vi ".....FACE RECOGNITION only.vi"() -> ()   [LabVIEW 2018]
doc: "This example shows how to use the Lucas Kanade Pyramid motion estimation VI to track features in a sequence of images in NI Vision. The VI reads the frames from an AVI file and tracks user specified features in the image from frame to frame."
uses:
  <vilib>/University of Leeds/Kinesthesia Toolkit for Microsoft Kinect/_Polymorphic Configure/Event-Video.vi
  <vilib>/University of Leeds/Kinesthesia Toolkit for Microsoft Kinect/_Polymorphic Read/Read-Video.vi
  <vilib>/University of Leeds/Kinesthesia Toolkit for Microsoft Kinect/_Polymorphic Close/Close-Video.vi
  <vilib>/vision/NI_Vision_Development_Module.lvlib
panel:
  out "Lips Template":T1(plugin-control)
  out "Nose Template":T1(plugin-control)
  out "Eye Template":T1(plugin-control)
  in  "Eye Min Score":sgl=700.0
  in  "Nose Min Score":sgl=700.0
  in  "Lip Min Score":sgl=700.0
  out "Preview":T1(plugin-control)
  in  "Show Templates":bool
  out "Face Found":bool
  # "Face Recognition System"
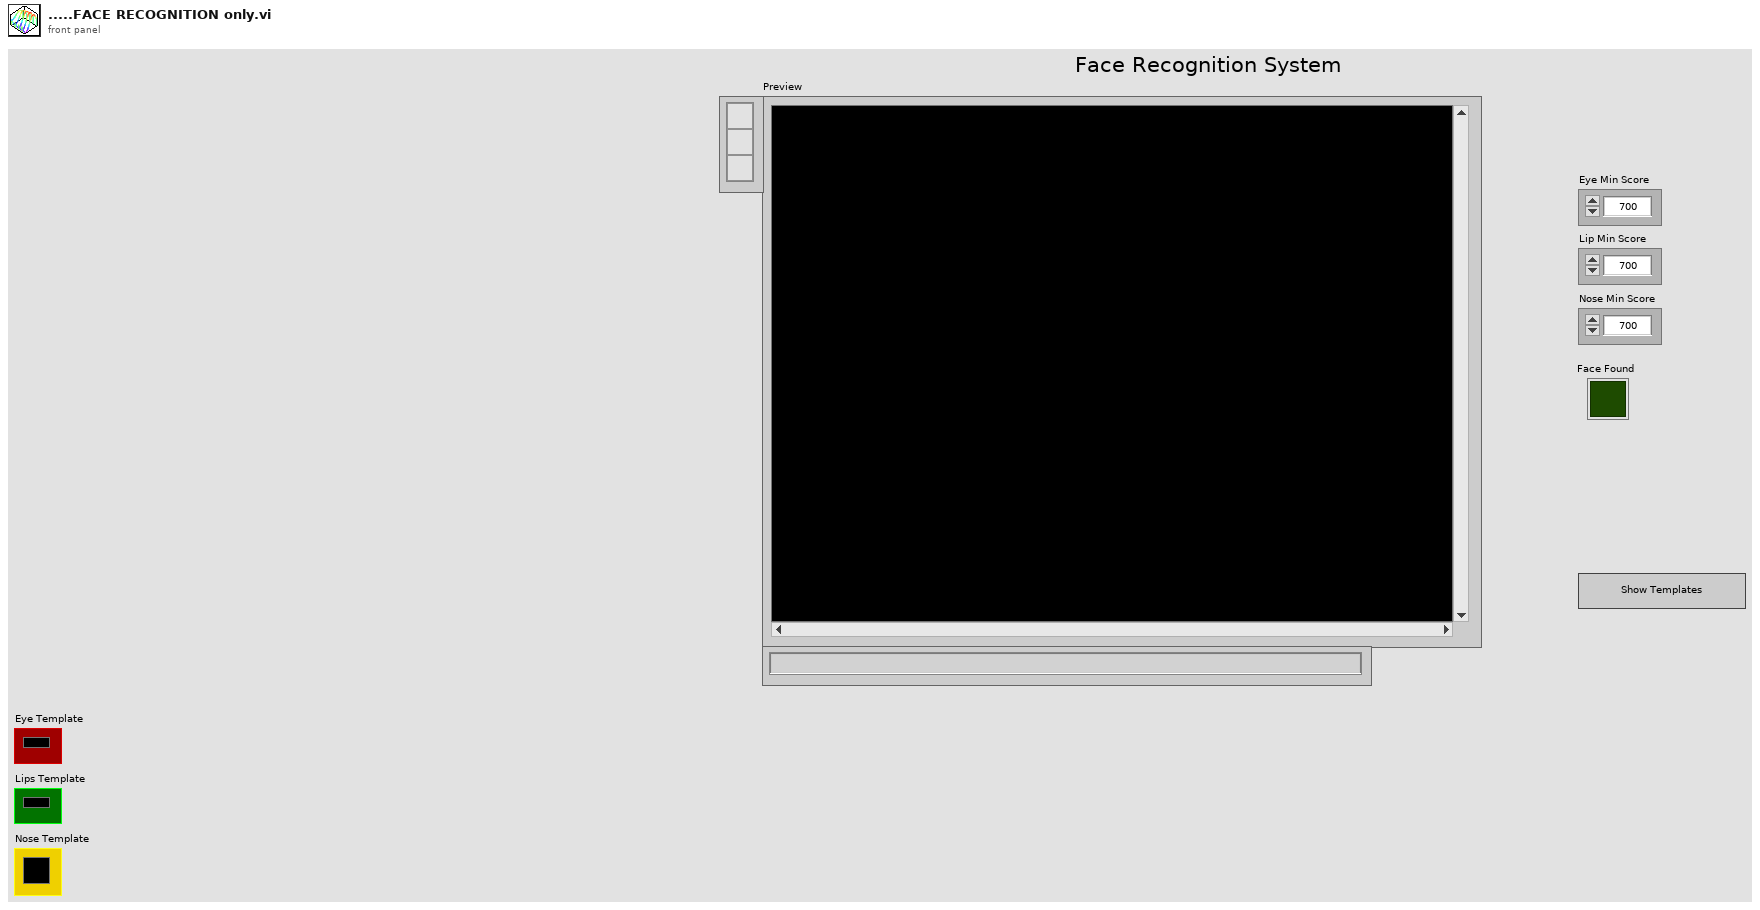
[diagram p1: front panel]
types:
  T1 = typedef "IMAQ Image.ctl" = refnum<image>
  T2 = cluster{cluster{"reference out":refnum<k24>, "KinectSensors":refnum<k24>}, "get_Item":refnum<k24>}
  T3 = cluster{"reference out":refnum<k24>, "KinectSensors":refnum<k24>, "ColorStream":refnum<k24>, "get_Item":refnum<k24>}
  T4 = typedef "Image Type" = u32
  T5 = cluster{"Position":cluster{"x":sgl, "y":sgl}, "Angle":sgl, "Scale":sgl, "Score":sgl, "Bounding Box":cluster{"x":sgl, "y":sgl}[]}[]
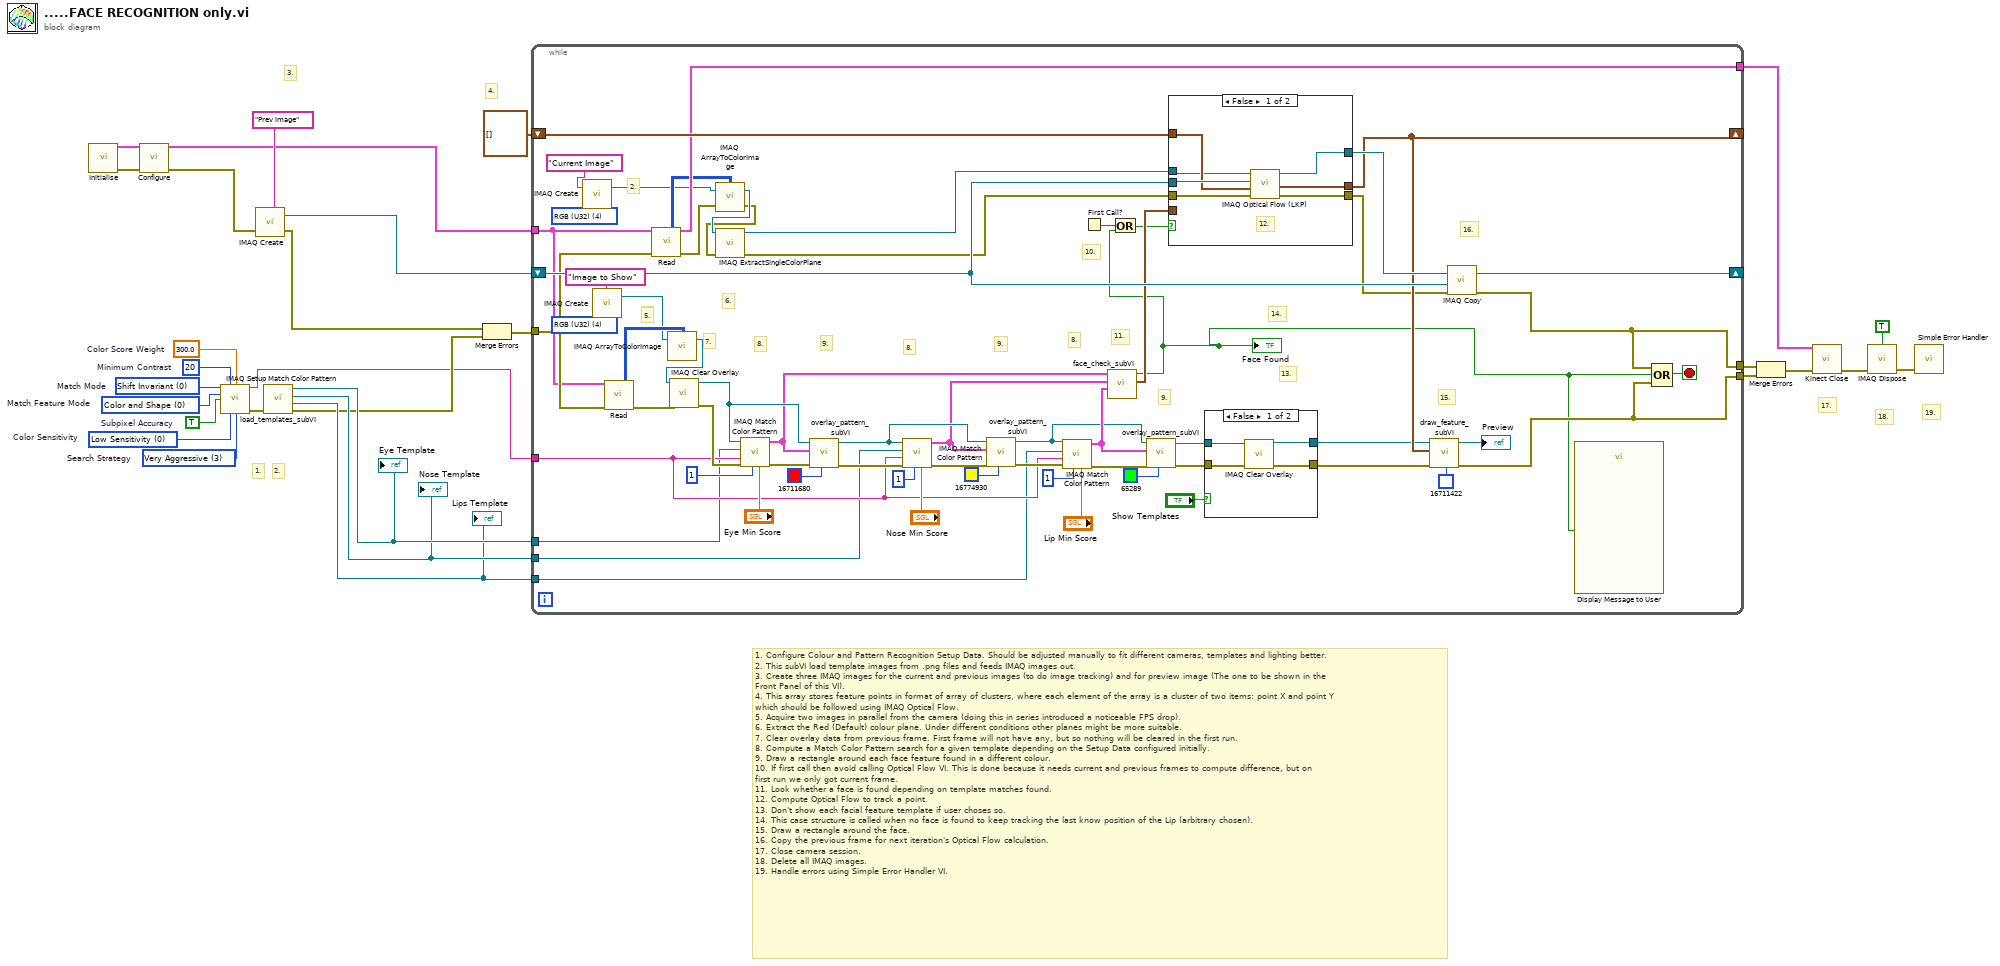
[diagram p0: block diagram]
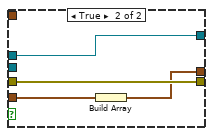
[diagram p3: hidden frame]
diagram:
  w16 = TRUE  # Subpixel Accuracy
  w22 = u32 0 items=["Color and Shape", "Color", "Shape"]  # Match Feature Mode
  w21 = u32 3 items=["Conservative", "Balance", "Aggressive", "Very Aggressive"]  # Search Strategy
  w20 = 20  # Minimum Contrast
  w19 = sgl 300.0  # Color Score Weight
  w18 = u32 0 items=["Low Sensitivity", "Medium Sensitivity", "High Sensitivity"]  # Color Sensitivity
  w17 = u32 0 items=["Shift Invariant", "Rotation Invariant"]  # Match Mode
  # "1. Configure Colour and Pattern Recognition Setup Data. Should be adjusted manually to fit different cameras, templates and lighting better.\n2. This subVI load template images from .png files and feeds IMAQ images out.\n3. Create three IMAQ images for the current and previous images (to do image tracking) and for preview image (The one to be shown in the\nFront Panel of this VI).\n4. This array stores feature points in format of array of clusters, where each element of the array is a cluster of two items: point X and point Y \nwhich should be followed using IMAQ Optical Flow.\n5. Acquire two images in parallel from the camera (doing this in series introduced a noticeable FPS drop).\n6. Extract the Red (Default) colour plane. Under different conditions other planes might be more suitable.\n7. Clear overlay data from previous frame. First frame will not have any, but so nothing will be cleared in the first run.\n8. Compute a Match Color Pattern search for a given template depending on the Setup Data configured initially.\n9. Draw a rectangle around each face feature found in a different colour.\n10. If first call then avoid calling Optical Flow VI. This is done because it needs current and previous frames to compute difference, but on\nfirst run we only got current frame.\n11. Look whether a face is found depending on template matches found.\n12. Compute Optical Flow to track a point.\n13. Don't show each facial feature template if user choses so.\n14. This case structure is called when no face is found to keep tracking the last know position of the Lip (arbitrary chosen).\n15. Draw a rectangle around the face.\n16. Copy the previous frame for next iteration's Optical Flow calculation.\n17. Close camera session.\n18. Delete all IMAQ images.\n19. Handle errors using Simple Error Handler VI."
  # "19."
  # "17."
  # "4."
  # "3."
  # "3."
  # "3."
  # "2."
  # "1."
  # "18."
  n1 = call <vilib>:"Initialise.vi"() -> ("Kinect References out"=w27:T2, "error out"=w26:errorcluster)  [unwired: 14 in]
  n2 = call-poly <vilib>:"Configure.vi"("Kinect References in"=w27, "error in"=w26) -> ("Kinect References out"=w23:T3, "error out"=w2:errorcluster)  [unwired: 12 in]
  n3 = call "IMAQ Setup Match Color Pattern"("Match Mode"=w17, "Minimum Contrast"=w20, "Color Score Weight"=w19, "Match Feature Mode"=w22, "Subpixel Accuracy"=w16, "Color Sensitivity"=w18, "Search Strategy"=w21) -> ("Match Color Pattern Setup Data"=w6:string, "error out"=w15:errorcluster)  [unwired: 7 in]
  n4 = call "IMAQ Create"("Image Name"="Prev Image", "error in (no error)"=w2) -> ("New Image"=w24:T1, "error out"=w1:errorcluster)  [unwired: 2 in, 1 out]
  n5 = call "load_templates_subVI.vi"("error in (no error)"=w15) -> ("error out"=w8:errorcluster, "Lips Template"=w12:T1, "Nose Template"=w13:T1, "Eye Template"=w14:T1)  [unwired: 7 in]
  "Eye Template" <- w14
  "Nose Template" <- w13
  "Lips Template" <- w12
  n6 = Merge Errors(w1, w8) -> (w7:errorcluster)
  n7 = while {
    shift-right: [w91] -> _
    shift-left: w24 -> [w92]
    shift-right: [w57] -> _
    shift-left: cluster{"X":sgl, "Y":sgl}[] [] ("Feature Points Out") -> [w90]
    tunnel: w23 -> [w48]
    tunnel: [w89] -> w28
    tunnel: w6 -> [w64]
    tunnel: w14 -> [w63]
    tunnel: w13 -> [w62]
    tunnel: w12 -> [w61]
    tunnel: w7 -> [w50]
    tunnel: [w46] -> w5
    tunnel: [w45] -> w4
    stop <- w47 stop-if-true
    w32 = T4 4 items=["Grayscale (U8)", "Grayscale (I16)", "Grayscale (SGL)", "Complex (CSG)", "RGB (U32)", "HSL (U32)", "RGB (U64)", "Grayscale (U16)"] ("Image Type")
    w34 = T4 4 items=["Grayscale (U8)", "Grayscale (I16)", "Grayscale (SGL)", "Complex (CSG)", "RGB (U32)", "HSL (U32)", "RGB (U64)", "Grayscale (U16)"] ("Image Type")
    # "4."
    # "2."
    # "10."
    # "16."
    # "15."
    # "14."
    # "13."
    # "11."
    # "9."
    # "8."
    # "9."
    # "8."
    # "9."
    # "8."
    # "7."
    # "6."
    # "5."
    # "5."
    n8 = call "IMAQ Create"("Image Name"="Current Image", "Image Type"=w32) -> ("New Image"=w36:T1)  [unwired: 2 in, 2 out]
    n9 = call "IMAQ Create"("Image Name"="Image to Show", "Image Type"=w34) -> ("New Image"=w31:T1)  [unwired: 2 in, 2 out]
    n10 = call-poly <vilib>:"Read.vi"("Kinect References in"=w48, "error in (no error)"=w50) -> ("Colour output array (U24, RGB)"=w40:u32[][], "error out"=w59:errorcluster)  [unwired: 10 in, 2 out]
    n11 = call-poly <vilib>:"Read.vi"("Kinect References in"=w48, "error in (no error)"=w50) -> ("Colour output array (U24, RGB)"=w42:u32[][], "Kinect References out"=w89:T3, "error out"=w38:errorcluster)  [unwired: 10 in, 1 out]
    n12 = call "IMAQ ArrayToColorImage"("Image Pixels (U32)"=w40, "Image"=w31) -> ("Image Out"=w39:T1)  [unwired: 3 in, 1 out]
    n13 = call "IMAQ Clear Overlay"("error in (no error)"=w59, "Image"=w39) -> ("error out"=w85:errorcluster, "Image Out"=w71:T1)  [unwired: 8 in]
    n14 = call "IMAQ ArrayToColorImage"("Image Pixels (U32)"=w42, "Image"=w36, "error in (no error)"=w38) -> ("Image Out"=w41:T1, "error out"=w37:errorcluster)  [unwired: 2 in]
    n15 = call "IMAQ ExtractSingleColorPlane"("error in (no error)"=w37, "Image Src"=w41) -> ("error out"=w88:errorcluster, "Image Dst Out"=w87:T1)  [unwired: 8 in]
    n16 = call "IMAQ Match Color Pattern"("Minimum Match Score"="Eye Min Score", "Number of Matches Requested"=1, "error in (no error)"=w85, "Match Color Pattern Setup Data"=w64, "Template Image"=w63, "Image"=w71) -> ("error out"=w84:errorcluster, "Matches"=w68:T5)  [unwired: 3 in, 1 out]
    n17 = call "overlay_pattern_subVI.vi"("Color"=u32 16711680, "error in"=w84, "Matches"=w68, "Image"=w71) -> ("error out"=w81:errorcluster, "Image Out"=w78:T1)  [unwired: 6 in]
    n18 = call "IMAQ Match Color Pattern"("Minimum Match Score"="Nose Min Score", "Number of Matches Requested"=1, "error in (no error)"=w81, "Match Color Pattern Setup Data"=w64, "Template Image"=w62, "Image"=w78) -> ("error out"=w79:errorcluster, "Matches"=w67:T5)  [unwired: 3 in, 1 out]
    n19 = call "overlay_pattern_subVI.vi"("Color"=u32 16774930, "error in"=w79, "Matches"=w67, "Image"=w78) -> ("error out"=w77:errorcluster, "Image Out"=w65:T1)  [unwired: 6 in]
    n20 = call "IMAQ Match Color Pattern"("Minimum Match Score"="Lip Min Score", "Number of Matches Requested"=1, "error in (no error)"=w77, "Match Color Pattern Setup Data"=w64, "Template Image"=w61, "Image"=w65) -> ("error out"=w76:errorcluster, "Matches"=w66:T5)  [unwired: 3 in, 1 out]
    n21 = First Call?() -> (First Call?: T/F=w43:bool)
    n22 = call "face_check_subVI.vi"("Lips Match"=w66, "Nose Match"=w67, "Eye Match"=w68) -> ("Lip Position"=w60:cluster{"x":sgl, "y":sgl}, "Face Found"=w30:bool)  [unwired: 6 in, 1 out]
    "Face Found" <- w30
    n23 = Or(x=w43, y=w30) -> (x .or. y?=w44:bool)
    n24 = call "overlay_pattern_subVI.vi"("Color"=u32 65289, "error in"=w76, "Matches"=w66, "Image"=w65) -> ("error out"=w53:errorcluster, "Image Out"=w55:T1)  [unwired: 6 in]
    n25 = case shown="False" w44 {
      tunnel: w92 -> [w105 _]
      tunnel: w90 -> [w104 _]
      tunnel: [w103 w106] -> w57
      tunnel: w88 -> [w102 w109]
      tunnel: w87 -> [w99 w108]
      tunnel: [w101 w108] -> w86
      tunnel: [w100 w109] -> w49
      tunnel: w60 -> [_ w107]
      frame False {
        # "12."
        n26 = call "IMAQ Optical Flow (LKP)"("error in (no error)"=w102, "Feature Points In"=w104, "Previous Frame"=w105, "Current Frame"=w99) -> ("error out"=w100:errorcluster, "Feature Points Out"=w103:cluster{"X":sgl, "Y":sgl}[], "Current Frame Out (dup)"=w101:T1)  [unwired: 2 in, 3 out]
      }
      frame True {
        n27 = Build Array(w107) -> (w106:cluster{"x":sgl, "y":sgl}[])
      }
    }
    n28 = case shown="False" "Show Templates" {
      tunnel: w55 -> [w96 w98]
      tunnel: [w95 w98] -> w54
      tunnel: w53 -> [w94 w97]
      tunnel: [w93 w97] -> w51
      frame False {
        n29 = call "IMAQ Clear Overlay"("error in (no error)"=w94, "Image"=w96) -> ("error out"=w93:errorcluster, "Image Out"=w95:T1)  [unwired: 8 in]
      }
      frame True {
      }
    }
    n30 = call "draw_feature_subVI.vi"("Color"=u32 16711422, "Error In"=w51, "Feature Ponts"=w57, "Image"=w54) -> ("Error Out"=w45:errorcluster, "Image Out"=→"Preview":T1)  [unwired: 6 out]
    n31 = call "IMAQ Copy"("error in (no error)"=w49, "Image Dst"=w92, "Image Src"=w86) -> ("error out"=w46:errorcluster, "Image Dst Out"=w91:T1)  [unwired: 3 out]
    n32 = call "Display Message to User"("Enable"=w30) -> ()  [unwired: 9 in, 2 out]
    n33 = Compound Arithmetic op=OR(w46, w30, w45) -> (w47:bool)
  }
  n34 = Merge Errors(w5, w4) -> (w3:errorcluster)
  n35 = call-poly <vilib>:"Kinect Close.vi"("Kinect References in"=w28, "error in"=w3) -> ("error out"=w11:errorcluster)  [unwired: 13 in]
  n36 = call "IMAQ Dispose"("All Images? (No)"=TRUE, "error in (no error)"=w11) -> ("error out"=w10:errorcluster)  [unwired: 1 in, 3 out]
  n37 = call <vilib>:"Simple Error Handler.vi"("error in (no error)"=w10) -> ()  [unwired: 1 in, 8 out]
